vi "Convert Saved Status.vi"(2 "Container State":T1 caption="容器状态", 3 "Display State":T2={"Front Color"=1985280, "User Event"=refnum} caption="显示状态") -> (1 "Display State To Save":variant caption="待保存显示状态")   [LabVIEW 2013, in "IP Adresss Control.xctl"]
uses:
  IP Adresss Control.xctl
  IP Address Status.ctl
  UserEvent/IP User Event.ctl
  <vilib>/_xctls/Container State.ctl
  <vilib>/_xctls/XControlSupport.lvlib
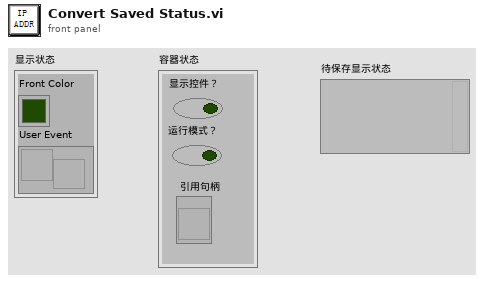
[diagram p1: front panel]
types:
  T1 = typedef "XControlSupport.lvlib/Container State.ctl" = cluster{"Indicator?":bool, "Run Mode?":bool, " Refnum":refnum<vi>}
  T2 = typedef "IP Adresss Control.xctl/IP Address Status.ctl" = cluster{"Front Color":u32, "User Event":refnum<user-event>}
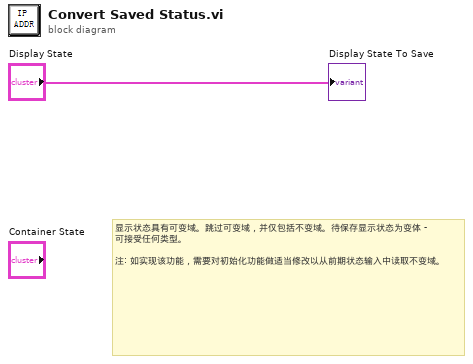
[diagram p0: block diagram]
diagram:
  # "显示状态具有可变域。跳过可变域，并仅包括不变域。待保存显示状态为变体 - 可接受任何类型。\n\n注: 如实现该功能，需要对初始化功能做适当修改以从前期状态输入中读取不变域。"
  "Display State To Save" <- "Display State"
